vi "Modem Status Command Answer Q.vi"(8 "error in (no error)":errorcluster) -> (0 "error out":errorcluster, 3 "notifier out":refnum<notifier>)   [LabVIEW 2011]
uses:
  Modem Status Raw Analog Data Cluster.ctl
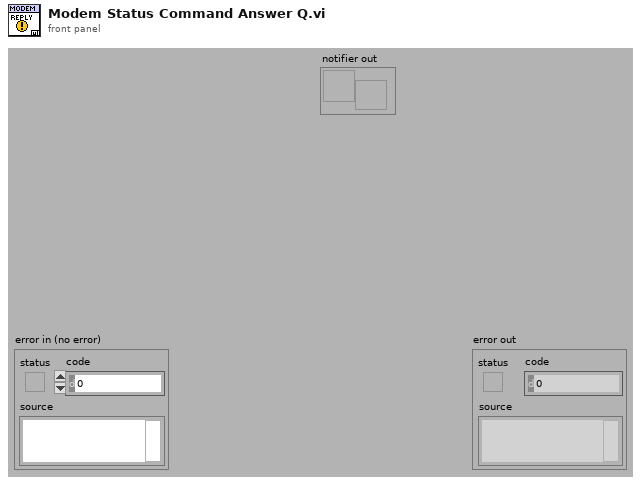
[diagram p1: front panel]
types:
  T1 = typedef "Modem Status Raw Analog Data Cluster.ctl" = cluster{"PCB Temp TS":dbl, "PCB Temp DH":dbl, "RX Gain TS":dbl, "RX Gain DH":dbl, "Signal Quality TS":dbl, "Signal Quality DH":dbl, "Numeric Link Status":dbl, "Link Status":bool}
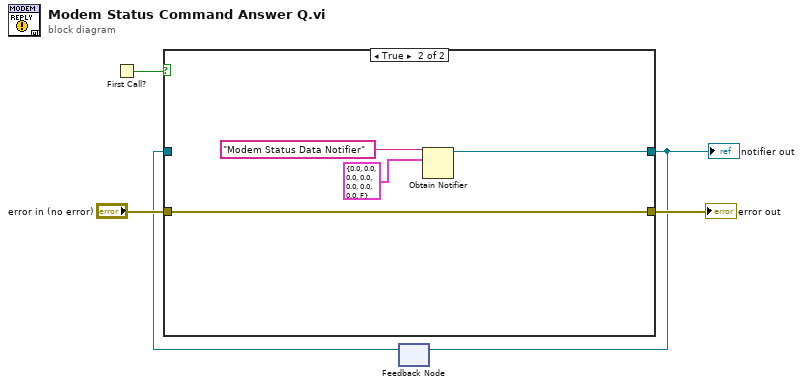
[diagram p0: block diagram]
diagram:
  n1 = First Call?() -> (First Call?: T/F=w3:bool)
  n2 = feedback #1() -> (w1:refnum<notifier>)  [unwired: 1 in]
  n3 = case shown="True" w3 {
    tunnel: [w7 w11] -> w5
    tunnel: "error in (no error)" -> [w7 w11]
    tunnel: [w6 w9] -> w2
    tunnel: w1 -> [w6 _]
    frame False {
    }
    frame True {
      n4 = Obtain Notifier(name (unnamed)="Modem Status Data Notifier", notification data type=T1 {"PCB Temp TS"=0.0, "PCB Temp DH"=0.0, "RX Gain TS"=0.0, "RX Gain DH"=0.0, "Signal Quality TS"=0.0, "Signal Quality DH"=0.0, "Numeric Link Status"=0.0, "Link Status"=FALSE} ("Modem Status Raw Analog Data Out")) -> (notifier out=w9:refnum<notifier>)  [unwired: 2 in, 2 out]
    }
  }
  "error out" <- w5
  "notifier out" <- w2
  n5 = feedback-in #1(w2) -> ()
